vi "Configure Power-on Defaults.vi"(8 "error in (no error)":errorcluster, 9 "Power Line Frequency (0: )":i32(ring) items=["", "50 Hz", "60 Hz"], 10 "Power-on Defaults (1: PreSet)":i32(ring)=1 items=["RST", "PreSet", "Save0", "Save1", "Save2", "Save3", "Save4", "Save5", "Save6", "Save7", "Save8", "Save9"], 11 "VISA resource name":refnum<visa-resource-name>) -> (0 "error out":errorcluster, 3 "VISA resource name out":refnum<visa-resource-name>)   [LabVIEW 2020, in "Keithley 6517.lvlib"]
doc: "Configures power-on defaults."
uses:
  <instrlib>/Keithley 6517/Keithley 6517.lvlib
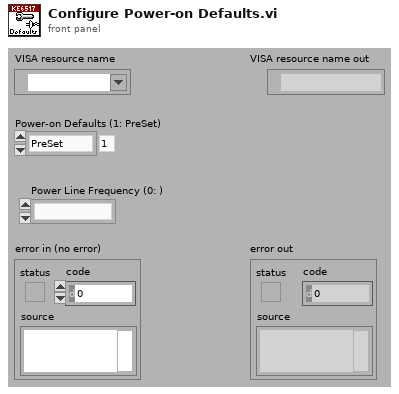
[diagram p1: front panel]
types:
  T1 = typedef "Keithley 6517.lvlib/Extended User Data.ctl" = cluster{"Instrument Model":i32}
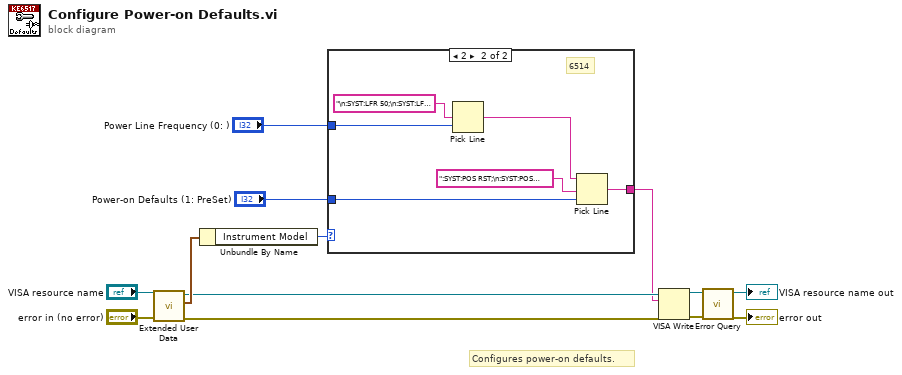
[diagram p0: block diagram]
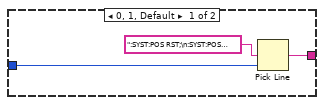
[diagram p2: hidden frame]
diagram:
  # "Configures power-on defaults."
  n1 = call <instrlib>:"Extended User Data.vi"("error in (no error)"="error in (no error)", "VISA resource name"="VISA resource name") -> ("error out"=w4:errorcluster, "User Data Out"=w8:T1, "VISA resource name out"=w3:refnum<visa-resource-name>)  [unwired: 7 in]
  n2 = Unbundle By Name(w8) -> ("Instrument Model"=w7:i32)
  n3 = case shown="2" w7 {
    tunnel: "Power-on Defaults (1: PreSet)" -> [w15 w21]
    tunnel: [w14 w20] -> w2
    tunnel: "Power Line Frequency (0: )" -> [_ w19]
    frame 0, 1, Default {
      n4 = Pick Line(multi-line string=":SYST:POS RST;\n:SYST:POS PRES;\n:SYST:POS SAV0;\n:SYST:POS SAV1;\n:SYST:POS SAV2;\n:SYST:POS SAV3;\n:SYST:POS SAV4;\n:SYST:POS SAV5;\n:SYST:POS SAV6;\n:SYST:POS SAV7;\n:SYST:POS SAV8;\n:SYST:POS SAV9;", line index=w15) -> (output string=w14:string)  [unwired: 1 in]
    }
    frame 2 {
      # "6514"
      n5 = Pick Line(multi-line string="\n:SYST:LFR 50;\n:SYST:LFR 60;", line index=w19) -> (output string=w18:string)  [unwired: 1 in]
      n6 = Pick Line(string ("")=w18, multi-line string=":SYST:POS RST;\n:SYST:POS PRES;\n:SYST:POS SAV0;\n:SYST:POS SAV1;\n:SYST:POS SAV2;\n:SYST:POS SAV3;\n:SYST:POS SAV4;", line index=w21) -> (output string=w20:string)
    }
  }
  n7 = VISA Write(VISA resource name=w3, write buffer=w2, error in (no error)=w4) -> (VISA resource name out=w13:refnum<visa-resource-name>, error out=w12:errorcluster)  [unwired: 1 out]
  n8 = call <instrlib>:"Error Query.vi"("error in (no error)"=w12, "VISA resource name"=w13) -> ("error out"=→"error out":errorcluster, "VISA resource name out"=→"VISA resource name out":refnum<visa-resource-name>)  [unwired: 6 in, 2 out]
